vi "Config Event Blender.vi"(0 "VISA resource name":refnum<visa-resource-name>, 1 "Input Event 1":string="0", 2 "Input Event 2":string="0", 3 "Input Event 3":string="0", 5 "Node In":string, 7 "Blender Number (1)":u32=1 min=1 max=4, 9 "Blend Type (OR)":enum16{"OR", "AND"}(ring), 11 "error in":errorcluster, 12 "Input Event 4":string="0") -> (4 "VISA resource name out":refnum<visa-resource-name>, 6 "Node Out":string, 14 "Command String":string, 15 "error out":errorcluster)   [LabVIEW 2018, in "Keithley 2600 Series.lvlib"]
doc: "This VI configures an event blender in the advanced trigger module.\n\n<b>Functions and Attributes Used</b>\ntrigger.blender[n].orenable\ntrigger.blender[n1].stimulus[n2]"
uses:
  Keithley 2600 Series.lvlib
  Private/GlobalVariables.vi
panel:
  # "(c) 2008 Keithley Instruments, Inc.  ALL RIGHTS RESERVED."
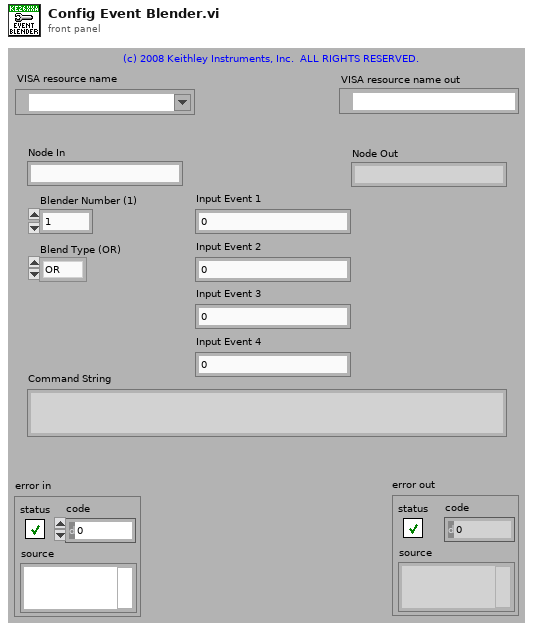
[diagram p1: front panel]
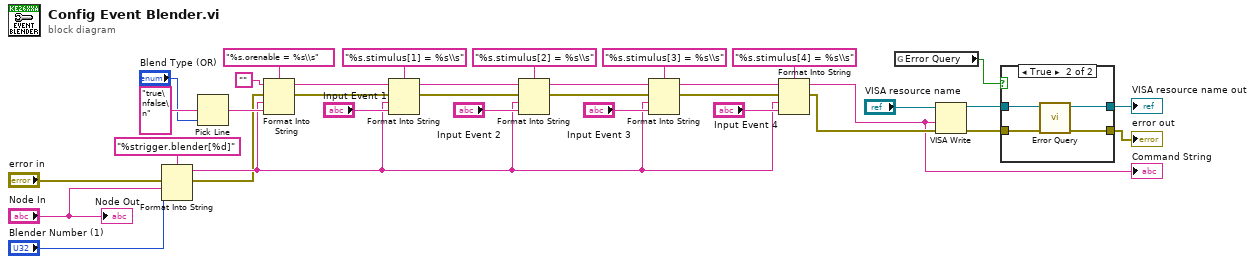
[diagram p0: block diagram]
diagram:
  n1 = Format Into String(format string="%strigger.blender[%d]", error in="error in", "Node In", "Blender Number (1)") -> (resulting string=w15:string, error out=w14:errorcluster)  [unwired: 1 in]
  n2 = Pick Line(multi-line string="true\nfalse\n", line index="Blend Type (OR)") -> (output string=w24:string)  [unwired: 1 out]
  n3 = Format Into String(format string="%s.orenable = %s\\s", initial string="", error in=w14, w15, w24) -> (resulting string=w5:string, error out=w19:errorcluster)
  n4 = Format Into String(format string="%s.stimulus[1] = %s\\s", initial string=w5, error in=w19, w15, "Input Event 1") -> (resulting string=w4:string, error out=w18:errorcluster)
  n5 = Format Into String(format string="%s.stimulus[2] = %s\\s", initial string=w4, error in=w18, w15, "Input Event 2") -> (resulting string=w3:string, error out=w17:errorcluster)
  n6 = Format Into String(format string="%s.stimulus[3] = %s\\s", initial string=w3, error in=w17, w15, "Input Event 3") -> (resulting string=w2:string, error out=w16:errorcluster)
  n7 = Format Into String(format string="%s.stimulus[4] = %s\\s", initial string=w2, error in=w16, w15, "Input Event 4") -> (resulting string=w6:string, error out=w13:errorcluster)
  "Command String" <- w6
  n8 = global read "GlobalVariables.vi" "Error Query"() -> (w11:bool)
  n9 = VISA Write(VISA resource name="VISA resource name", write buffer=w6, error in (no error)=w13) -> (VISA resource name out=w10:refnum<visa-resource-name>, error out=w9:errorcluster)  [unwired: 1 out]
  n10 = case shown="True" w11 {
    tunnel: w10 -> [w37 w41]
    tunnel: w9 -> [w36 w40]
    tunnel: [w37 w39] -> w8
    tunnel: [w36 w38] -> w7
    frame False {
    }
    frame True {
      n11 = call "Error Query.vi"("error in (no error)"=w40, "VISA resource name"=w41) -> ("error out"=w38:errorcluster, "VISA resource name out"=w39:refnum<visa-resource-name>)  [unwired: 8 out]
    }
  }
  "VISA resource name out" <- w8
  "error out" <- w7
  "Node Out" <- "Node In"
